vi "HMAC.vi"(5 "Output length (-1)":i32=-1, 7 "HASH-method":T1=enum."SHA-256" caption="HASH-method (SHA-256)", 8 "error in (no error)":errorcluster, 10 "Key":u8[](array[numeric]), 11 "Message":u8[](array[numeric])) -> (0 "error out":errorcluster, 1 "ASCII Formatted digest":string, 3 "HMAC digest":u8[](array[numeric]))   [LabVIEW 2011, in "i3-external-encryption.lvlib"]
doc: "Calculates the HMAC bases on the <b>Message</b> and <b>Key</b>.\n\n(c) Ton Plomp, 2011\nTHIS SOFTWARE IS PROVIDED AS IS, AND ANY WARRANTY IS REJECTED"
uses:
  i3-external-encryption.lvlib
  hash-types.ctl
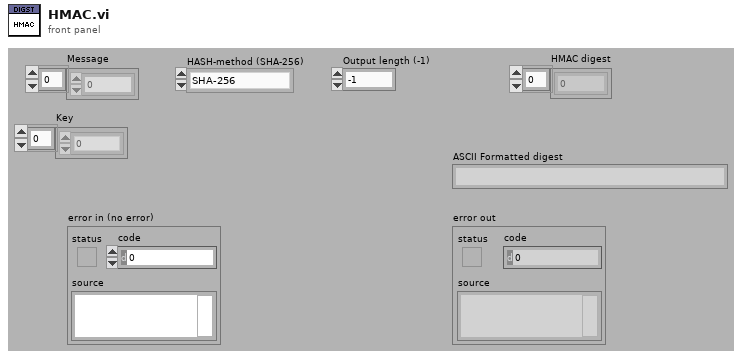
[diagram p1: front panel]
types:
  T1 = typedef "i3-external-encryption.lvlib/hash-types.ctl" = enum16{"MD5", "SHA-1", "SHA-224", "SHA-256", "SHA-384", "SHA-512"}
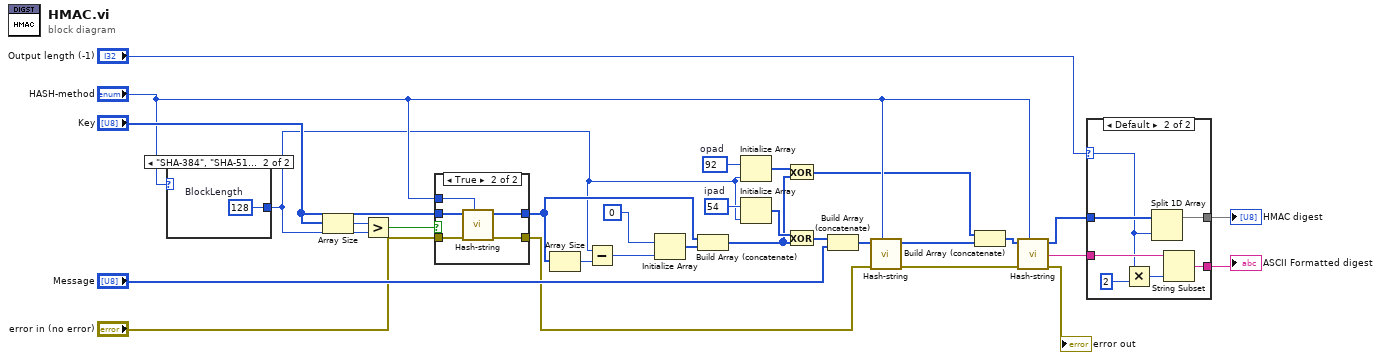
[diagram p0: block diagram]
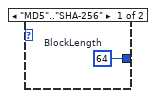
[diagram p4: hidden frame]
diagram:
  w25 = u8 92  # opad
  w30 = u8 54  # ipad
  n1 = case shown="\"SHA-384\", \"SHA-512\"" "HASH-method" {
    tunnel: [w31 w32] -> w4
    frame "MD5".."SHA-256" {
      w31 = 64  # BlockLength
    }
    frame "SHA-384", "SHA-512" {
      w32 = 128  # BlockLength
    }
  }
  n2 = Array Size(array="Key") -> (size(s)=w18:i32)
  n3 = Greater?(x=w18, y=w4) -> (0:w17:bool)
  n4 = case shown="True" w17 {
    tunnel: "Key" -> [w34 w35]
    tunnel: [w34 w36] -> w15
    tunnel: "HASH-method" -> [_ w39]
    tunnel: "error in (no error)" -> [w33 w38]
    tunnel: [w33 w37] -> w13
    frame False {
    }
    frame True {
      n5 = call "Hash-string.vi"("HASH-method"=w39, "error in (no error)"=w38, "Message"=w35) -> ("error out"=w37:errorcluster, "Hash"=w36:u8[])  [unwired: 6 in, 1 out]
    }
  }
  n6 = Array Size(array=w15) -> (size(s)=w29:i32)
  n7 = Subtract(x=w4, y=w29) -> (x-y=w28:i32)
  n8 = Initialize Array(u8 0, w28) -> (w27:u8[])
  n9 = Build Array (concatenate)(w15, w27) -> (w2:u8[])
  n10 = Initialize Array(w25, w4) -> (w24:u8[])
  n11 = Initialize Array(w30, w4) -> (w26:u8[])
  n12 = Exclusive Or(1:w2, 2:w24) -> (0:w5:u8[])
  n13 = Exclusive Or(1:w2, 2:w26) -> (0:w6:u8[])
  n14 = Build Array (concatenate)(w6, "Message") -> (w22:u8[])
  n15 = call "Hash-string.vi"("HASH-method"="HASH-method", "error in (no error)"=w13, "Message"=w22) -> ("error out"=w20:errorcluster, "Hash"=w1:u8[])  [unwired: 6 in, 1 out]
  n16 = Build Array (concatenate)(w5, w1) -> (w21:u8[])
  n17 = call "Hash-string.vi"("HASH-method"="HASH-method", "error in (no error)"=w20, "Message"=w21) -> ("error out"=→"error out":errorcluster, "ASCII formatted hash"=w10:string, "Hash"=w12:u8[])  [unwired: 6 in]
  n18 = case shown="Default" "Output length (-1)" {
    selector: "Output length (-1)" -> [_ w44]
    tunnel: w12 -> [w41 w48]
    tunnel: [w41 w42] -> w11
    tunnel: w10 -> [w40 w47]
    tunnel: [w40 w46] -> w9
    frame -1 {
    }
    frame Default {
      n19 = Multiply(x=w44, y=2) -> (x*y=w43:i32)
      n20 = Split 1D Array(array=w48, index=w44) -> (first subarray=w42:u8[])  [unwired: 1 out]
      n21 = String Subset(string=w47, length (rest)=w43) -> (substring=w46:string)  [unwired: 1 in]
    }
  }
  "HMAC digest" <- w11
  "ASCII Formatted digest" <- w9
